vi "LP01n.vi"() -> ()   [LabVIEW 2010]
panel:
  in  "?":i32=123
  in  "?":i32=123
  out "Сушилка":picture
  out "Датчик наличия рук":bool
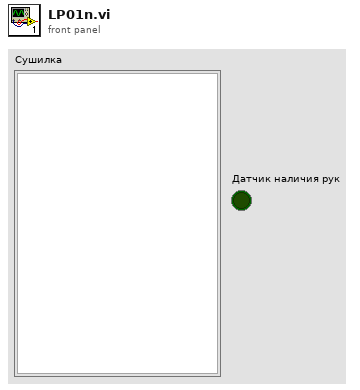
[diagram p1: front panel]
types:
  T1 = typedef "imagedata.ctl" = cluster{"image type":i32, "image depth":i32, "image":u8[], "mask":u8[], "colors":u32[], "Rectangle":cluster{"left":i16, "top":i16, "right":i16, "bottom":i16}}
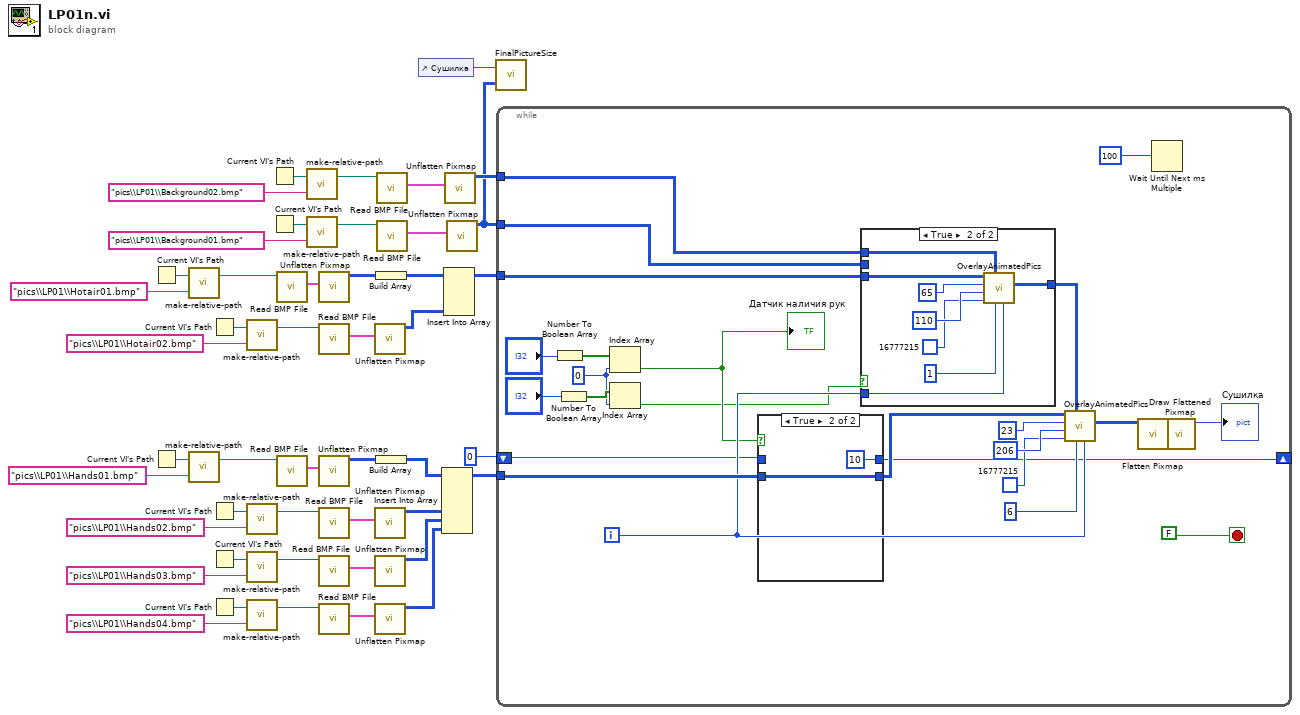
[diagram p0: block diagram]
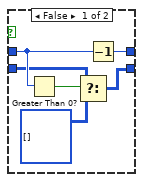
[diagram p2: hidden frame]
diagram:
  n1 = Current VI's Path() -> (path=w37:path)
  n2 = Current VI's Path() -> (path=w23:path)
  n3 = call "make-relative-path.vi"("Relative Path"="pics\\LP01\\Hotair01.bmp" ("name or relative path"), "the current VI's path"=w37) -> ("Constructed Path"=w38:path)  [unwired: 1 out]
  n4 = call "make-relative-path.vi"("Relative Path"="pics\\LP01\\Hands01.bmp" ("name or relative path"), "the current VI's path"=w23) -> ("Constructed Path"=w22:path)  [unwired: 1 out]
  n5 = Current VI's Path() -> (path=w41:path)
  n6 = Current VI's Path() -> (path=w19:path)
  n7 = Current VI's Path() -> (path=w12:path)
  n8 = Current VI's Path() -> (path=w7:path)
  n9 = call "make-relative-path.vi"("Relative Path"="pics\\LP01\\Hotair02.bmp" ("name or relative path"), "the current VI's path"=w41) -> ("Constructed Path"=w42:path)  [unwired: 1 out]
  n10 = call "make-relative-path.vi"("Relative Path"="pics\\LP01\\Hands02.bmp" ("name or relative path"), "the current VI's path"=w19) -> ("Constructed Path"=w18:path)  [unwired: 1 out]
  n11 = call "make-relative-path.vi"("Relative Path"="pics\\LP01\\Hands03.bmp" ("name or relative path"), "the current VI's path"=w12) -> ("Constructed Path"=w11:path)  [unwired: 1 out]
  n12 = call "make-relative-path.vi"("Relative Path"="pics\\LP01\\Hands04.bmp" ("name or relative path"), "the current VI's path"=w7) -> ("Constructed Path"=w6:path)  [unwired: 1 out]
  n13 = Current VI's Path() -> (path=w35:path)
  n14 = Current VI's Path() -> (path=w28:path)
  n15 = call <vilib>:"Read BMP File.vi"("path to BMP file"=w38) -> ("image data"=w39:T1)  [unwired: 8 in, 2 out]
  n16 = call <vilib>:"Read BMP File.vi"("path to BMP file"=w22) -> ("image data"=w21:T1)  [unwired: 8 in, 2 out]
  n17 = call "make-relative-path.vi"("Relative Path"="pics\\LP01\\Background02.bmp" ("name or relative path"), "the current VI's path"=w35) -> ("Constructed Path"=w34:path)  [unwired: 1 out]
  n18 = call "make-relative-path.vi"("Relative Path"="pics\\LP01\\Background01.bmp" ("name or relative path"), "the current VI's path"=w28) -> ("Constructed Path"=w27:path)  [unwired: 1 out]
  n19 = call <vilib>:"Unflatten Pixmap.vi"("image data"=w39) -> ("24-bit pixmap"=w44:u32[][])  [unwired: 4 in, 6 out]
  n20 = call <vilib>:"Read BMP File.vi"("path to BMP file"=w42) -> ("image data"=w43:T1)  [unwired: 8 in, 2 out]
  n21 = call <vilib>:"Unflatten Pixmap.vi"("image data"=w21) -> ("24-bit pixmap"=w16:u32[][])  [unwired: 4 in, 6 out]
  n22 = call <vilib>:"Read BMP File.vi"("path to BMP file"=w18) -> ("image data"=w17:T1)  [unwired: 8 in, 2 out]
  n23 = call <vilib>:"Read BMP File.vi"("path to BMP file"=w11) -> ("image data"=w10:T1)  [unwired: 8 in, 2 out]
  n24 = call <vilib>:"Read BMP File.vi"("path to BMP file"=w6) -> ("image data"=w5:T1)  [unwired: 8 in, 2 out]
  n25 = call <vilib>:"Unflatten Pixmap.vi"("image data"=w43) -> ("24-bit pixmap"=w46:u32[][])  [unwired: 4 in, 6 out]
  n26 = call <vilib>:"Unflatten Pixmap.vi"("image data"=w17) -> ("24-bit pixmap"=w14:u32[][])  [unwired: 4 in, 6 out]
  n27 = call <vilib>:"Unflatten Pixmap.vi"("image data"=w10) -> ("24-bit pixmap"=w9:u32[][])  [unwired: 4 in, 6 out]
  n28 = call <vilib>:"Unflatten Pixmap.vi"("image data"=w5) -> ("24-bit pixmap"=w4:u32[][])  [unwired: 4 in, 6 out]
  n29 = Build Array(w44) -> (w45:u32[][][])
  n30 = Build Array(w16) -> (w15:u32[][][])
  n31 = call <vilib>:"Read BMP File.vi"("path to BMP file"=w34) -> ("image data"=w33:T1)  [unwired: 8 in, 2 out]
  n32 = call <vilib>:"Read BMP File.vi"("path to BMP file"=w27) -> ("image data"=w26:T1)  [unwired: 8 in, 2 out]
  n33 = control-ref of="Сушилка"() -> (w2:refnum<vi>)
  n34 = Insert Into Array(array=w15, new element #1=w14, new element #2=w9, new element #3=w4) -> (w3:u32[][][])  [unwired: 3 in]
  n35 = Insert Into Array(array=w45, new element=w46) -> (w30:u32[][][])  [unwired: 3 in]
  n36 = call <vilib>:"Unflatten Pixmap.vi"("image data"=w33) -> ("24-bit pixmap"=w31:u32[][])  [unwired: 4 in, 6 out]
  n37 = call <vilib>:"Unflatten Pixmap.vi"("image data"=w26) -> ("24-bit pixmap"=w25:u32[][])  [unwired: 4 in, 6 out]
  n38 = call "FinalPictureSize.vi"("Background pixmap"=w25, "Link to final picture"=w2) -> ()
  n39 = while {
    tunnel: w31 -> [w62]
    tunnel: w30 -> [w61]
    tunnel: w25 -> [w60]
    tunnel: w3 -> [w59]
    shift-right: [w54] -> _
    shift-left: 0 -> [w55]
    i -> [w58]
    stop <- FALSE stop-if-true
    w47 = 0
    n40 = Number To Boolean Array(number="?") -> (Boolean array=w51:bool[])
    n41 = Number To Boolean Array(number="?") -> (Boolean array=w49:bool[])
    n42 = Index Array(array=w51, index=w47) -> (element=w50:bool)
    "Датчик наличия рук" <- w50
    n43 = Index Array(array=w49, index=w47) -> (element=w48:bool)
    n44 = case shown="True" w50 {
      tunnel: w59 -> [w75 w79]
      tunnel: [w74 w79] -> w63
      tunnel: w55 -> [w76 _]
      tunnel: [w77 10] -> w54
      frame False {
        n45 = Greater Than 0?(x=w76) -> (x > 0?=w73:bool)
        n46 = Select(t=w75, s=w73, f=u32[][][] [] ("initialized array")) -> (s? t:f=w74:u32[][][])
        n47 = Decrement(x=w76) -> (x-1=w77:i32)
      }
      frame True {
      }
    }
    n48 = case shown="True" w48 {
      tunnel: [w80 w82] -> w64
      tunnel: w62 -> [_ w88]
      tunnel: w58 -> [_ w84]
      tunnel: w61 -> [_ w81]
      tunnel: w60 -> [w80 _]
      frame False {
      }
      frame True {
        n49 = call "OverlayAnimatedPics.vi"("Index"=w84, "Divisor"=1, "Background Array"=w88, "Color"=u32 16777215, "Y"=110 ("Y 2"), "X"=65 ("X 2"), "Array"=w81) -> ("Final Array"=w82:u32[][])  [unwired: 4 in]
      }
    }
    n50 = call "OverlayAnimatedPics.vi"("Index"=w58, "Divisor"=6 ("y"), "Background Array"=w64, "Color"=u32 16777215, "Y"=206, "X"=23, "Array"=w63) -> ("Final Array"=w69:u32[][])  [unwired: 4 in]
    n51 = call <vilib>:"Flatten Pixmap.vi"("24-bit pixmap"=w69) -> ("image data"=w70:T1)  [unwired: 10 in]
    n52 = Wait Until Next ms Multiple(millisecond multiple=100) -> ()  [unwired: 1 out]
    n53 = call <vilib>:"Draw Flattened Pixmap.vi"("image data"=w70) -> ("new picture"=→"Сушилка":picture)  [unwired: 8 in]
  }
